vi "FlyWheelSim_Example.vi"() -> ()   [LabVIEW 2019]
uses:
  <vilib>/Rock Robotics/WPI/ThirdParty/JAS_Junk/TrajLib/TypeDef/DCMOTOR.CTL
  <vilib>/Rock Robotics/WPI/ThirdParty/JAS_Junk/TrajLib/TypeDef/LINEAR_SYSTEM.ctl
  <vilib>/Analysis/Matrix/Datatypes/RealMatrix.ctl
  <vilib>/Rock Robotics/WPI/ThirdParty/JAS_Junk/TrajLib/TypeDef/LINEAR_QUADRATIC_REGULATOR.ctl
  <vilib>/Rock Robotics/WPI/ThirdParty/JAS_Junk/TrajLib/TypeDef/KALMAN_FILTER.ctl
  <vilib>/Rock Robotics/WPI/ThirdParty/JAS_Junk/TrajLib/TypeDef/LINEAR_SYSTEM_LOOP.ctl
  <vilib>/Rock Robotics/WPI/ThirdParty/JAS_Junk/TrajLib/TypeDef/LINEAR_PLANT_INV_FF.ctl
  <vilib>/Rock Robotics/WPI/ThirdParty/JAS_Junk/TrajLib/TypeDef/FLYWHEEL_SIM.ctl
  <vilib>/Rock Robotics/WPI/ThirdParty/JAS_Junk/TrajLib/TypeDef/LINEAR_SYSTEM_SIM.ctl
  <vilib>/Rock Robotics/WPI/ThirdParty/JAS_Junk/TrajLib/Enum/DCMOTOR_TYPES_ENUM.ctl
  <vilib>/Rock Robotics/WPI/ThirdParty/JAS_Junk/TrajLib/DCMotor_GetCIM.vi
  <vilib>/Rock Robotics/WPI/ThirdParty/JAS_Junk/TrajLib/DCMotor_GetAndymark9015.vi
  <vilib>/Rock Robotics/WPI/ThirdParty/JAS_Junk/TrajLib/DCMotor_GetAndymarkRs775_125.vi
  <vilib>/Rock Robotics/WPI/ThirdParty/JAS_Junk/TrajLib/DCMotor_GetBag.vi
  <vilib>/Rock Robotics/WPI/ThirdParty/JAS_Junk/TrajLib/DCMotor_GetBanebotsRs550.vi
  <vilib>/Rock Robotics/WPI/ThirdParty/JAS_Junk/TrajLib/DCMotor_GetBanebotsRs775.vi
  <vilib>/Rock Robotics/WPI/ThirdParty/JAS_Junk/TrajLib/DCMotor_GetFalcon500.vi
  <vilib>/Rock Robotics/WPI/ThirdParty/JAS_Junk/TrajLib/DCMotor_GetMiniCIM.vi
  <vilib>/Rock Robotics/WPI/ThirdParty/JAS_Junk/TrajLib/DCMotor_GetNEO.vi
  <vilib>/Rock Robotics/WPI/ThirdParty/JAS_Junk/TrajLib/DCMotor_GetNEO550.vi
  <vilib>/Rock Robotics/WPI/ThirdParty/JAS_Junk/TrajLib/DCMotor_GetRomiBuiltIn.vi
  <vilib>/Rock Robotics/WPI/ThirdParty/JAS_Junk/TrajLib/DCMotor_GetVex775Pro.vi
  <vilib>/Rock Robotics/WPI/ThirdParty/JAS_Junk/TrajLib/MatBuilder_Create.vi
  <vilib>/Rock Robotics/WPI/ThirdParty/JAS_Junk/TrajLib/LinearSystem_New.vi
  <vilib>/Rock Robotics/WPI/ThirdParty/JAS_Junk/TrajLib/MatrixHelper_Zero.vi
  <vilib>/Rock Robotics/WPI/ThirdParty/JAS_Junk/TrajLib/MatBuilder_Fill.vi
  <vilib>/Rock Robotics/WPI/ThirdParty/JAS_Junk/TrajLib/Matrix_Ident.vi
  <vilib>/Rock Robotics/WPI/ThirdParty/JAS_Junk/TrajLib/DCMotor_New.vi
  <vilib>/Rock Robotics/WPI/ThirdParty/JAS_Junk/TrajLib/MatrixHelper_CoerceSize.vi
  <vilib>/Analysis/7linalg.llb/Create Special Matrix.vi
  <vilib>/Analysis/7linalg.llb/Create Special Real Matrix.vi
  <vilib>/Rock Robotics/WPI/ThirdParty/JAS_Junk/TrajLib/Trajectory_Library.lvlib
  <vilib>/Analysis/Matrix/NI_Matrix.lvlib
panel:
  in  "Tab Control":T1(tab)
  out "Motor Current":dbl format="%20.3f"
  out "Battery Voltage":dbl format="%20.3f"
  in  "Shoot ball":bool
  out "CO Chart":cluster{dbl, "Voltage":dbl}(graph)
  in  "Shooter On/Off":bool
  out "Encoer Speed\nRad/Sec":dbl(slide) scale=0.0..300.0
  out "Speed":dbl format="%20.3f"
  out "Cor Err":bool
  out "Kalman Filtered\nSpeed":dbl format="%20.3f"
  out "PV Chart":T2(graph)
  out "Predict Err":bool
  out "Motor Volt Dmd (CO)":dbl format="%20.3f"
  out "shoot Start":bool
  out "Shoot Done":bool
  out "Shooter Motor":T3 {"Jr_KgM2" format="%13.5p"; "L_H" format="%13.5p"; "Kt_NMPerAmp" format="%13.5p"; "KvINV_RadPerSecPerVolt" format="%13.5p"; "R_Ohms" format="%13.5p"; "FreeSpeed_RadPerSec" format="%13.5p"; "FreeCurrent_Amps" format="%13.5p"; "StallCurrent_Amps" format="%13.5p"; "StallTorque_NM" format="%13.5p"; "nominalVoltage_Volts" format="%13.5p"}
  out "m_flywheelPlant_ALT":T4
  out "m_FlyWheelSim":T6 {"GearBox"."Jr_KgM2" format="%13.5p"; "GearBox"."L_H" format="%13.5p"; "GearBox"."Kt_NMPerAmp" format="%13.5p"; "GearBox"."KvINV_RadPerSecPerVolt" format="%13.5p"; "GearBox"."R_Ohms" format="%13.5p"; "GearBox"."FreeSpeed_RadPerSec" format="%13.5p"; "GearBox"."FreeCurrent_Amps" format="%13.5p"; "GearBox"."StallCurrent_Amps" format="%13.5p"; "GearBox"."StallTorque_NM" format="%13.5p"; "GearBox"."nominalVoltage_Volts" format="%13.5p"}
  out "Shooting A":T5
  out "Shooting B":T5
  out "KalmanFilter":T8
  out "Kalman Error":errorcluster
  out "LinearQuadraticRegulator":T9
  out "LQR Error":bool
  out "Linear System Loop":T10
  out "LinSysLoop_Error":bool
  # "<States,States>"
  # "<States,Inputs>"
  # "<Outputs,States>"
  # "<Outputs,Inputs>"
  # "<States, 1>"
  # "<Outputs, 1>"
  # "<Inputs, 1>"
  # "<Outputs, 1>"
  # "<States,States>"
  # "<States,Inputs>"
  # "<Outputs,States>"
  # "<Outputs,Inputs>"
  # "Steady State Gain  \n<States,Outputs>"
  # "State Estimate <Statess,1>"
  # "<States,States>"
  # "<States,Inputs>"
  # "<Outputs,States>"
  # "<Outputs,Inputs>"
  # "Ref State <States,1>"
  # "Comp and capped \noutput <Inputs,1>"
  # "Controller gain\n<Inputs,States>"
  # "<States,1>"
  # "<FUTURE --- CLAMP TYPE -- For now\nuse Normalize>"
  # "Steady State Gain  \n<States,Outputs>"
  # "State Estimate <Statess,1>"
  # "<States,States>"
  # "<States,Inputs>"
  # "<Outputs,States>"
  # "<Outputs,Inputs>"
  # "<States,1>"
  # "<Inputs,1>"
  # "<States,Inputs>"
  # "<States,States>"
  # "Ref State <States,1>"
  # "Comp and capped \noutput <Inputs,1>"
  # "Controller gain\n<Inputs,States>"
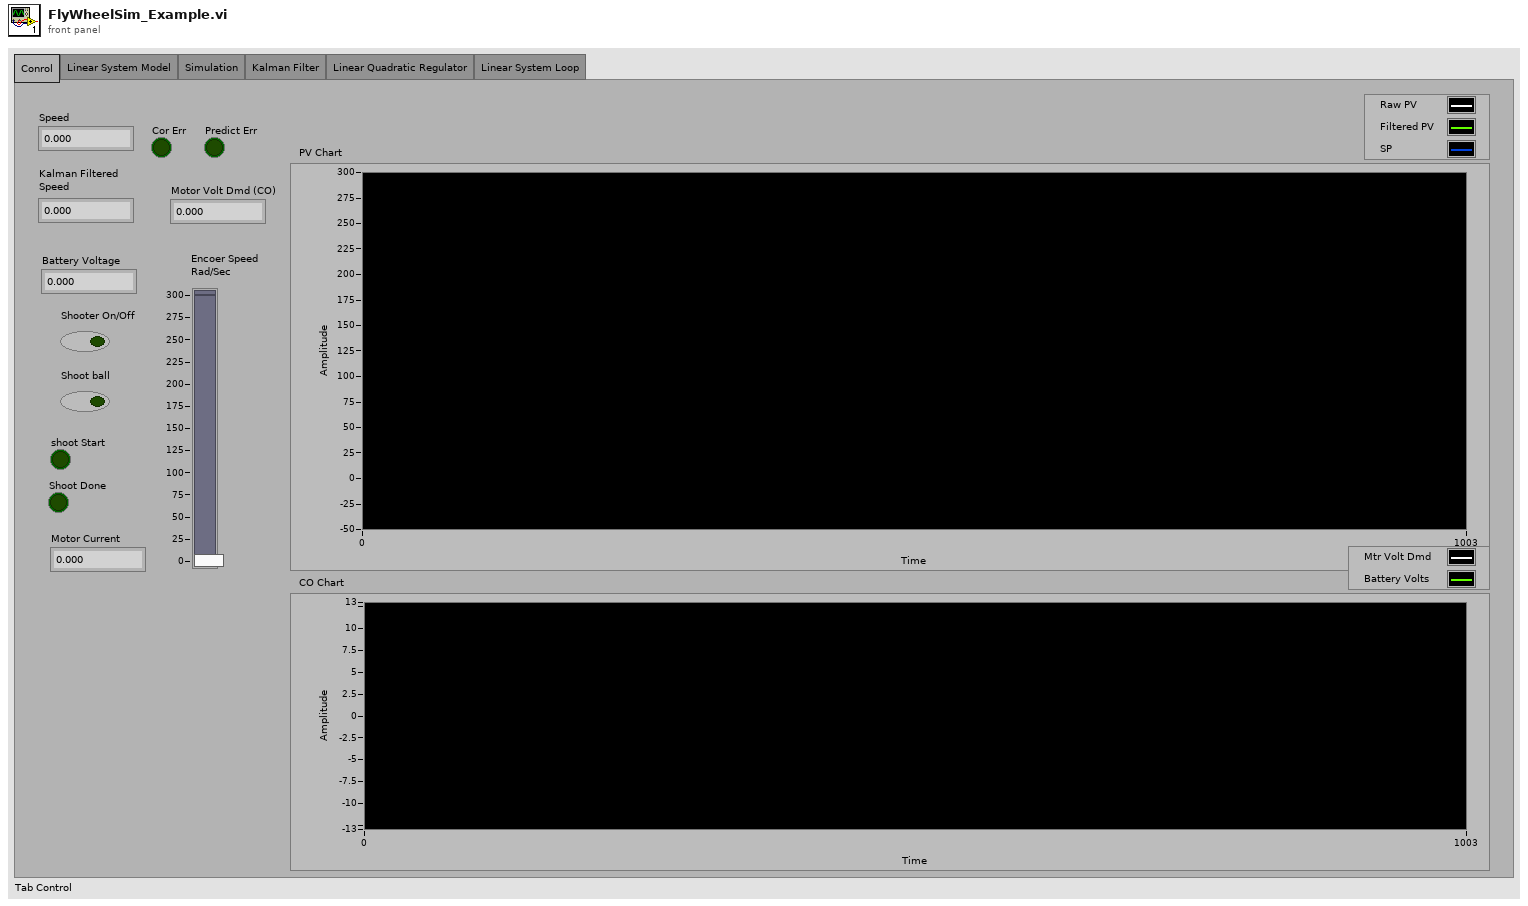
[diagram p1: front panel]
types:
  T1 = enum32{"Conrol", "Linear System Model", "Simulation", "Kalman Filter", "Linear Quadratic Regulator", "Linear System Loop"}
  T2 = cluster{"upper limit":dbl, "Real Matrix Element":dbl, "Real Matrix Element":dbl}
  T3 = typedef "Trajectory_Library.lvlib/DCMOTOR.CTL" = cluster{"nominalVoltage_Volts":dbl, "StallTorque_NM":dbl, "StallCurrent_Amps":dbl, "FreeCurrent_Amps":dbl, "FreeSpeed_RadPerSec":dbl, "R_Ohms":dbl, "KvINV_RadPerSecPerVolt":dbl, "Kt_NMPerAmp":dbl, "L_H":dbl, "Jr_KgM2":dbl}
  T4 = typedef "Trajectory_Library.lvlib/LINEAR_SYSTEM.ctl" = cluster{"m_A":T5, "m_B":T5, "m_C":T5, "m_D":T5, "States":i32, "Inputs":i32, "Outputs":i32}
  T5 = typedef "NI_Matrix.lvlib/RealMatrix.ctl" = dbl[][]
  T6 = typedef "Trajectory_Library.lvlib/FLYWHEEL_SIM.ctl" = cluster{"LinearSystemSim":T7, "GearBox":T3, "Gearing":dbl}
  T7 = typedef "Trajectory_Library.lvlib/LINEAR_SYSTEM_SIM.ctl" = cluster{"m_Plant":T4, "m_X":T5, "m_Y":T5, "m_U":T5, "MeasureStdDev":T5}
  T8 = typedef "Trajectory_Library.lvlib/KALMAN_FILTER.ctl" = cluster{"m_K":T5, "m_xHat":T5, "States":i32, "Outputs":i32, "m_Plant":T4}
  T9 = typedef "Trajectory_Library.lvlib/LINEAR_QUADRATIC_REGULATOR.ctl" = cluster{"m_r":T5, "m_U":T5, "m_K":T5, "States":i32, "Inputs":i32}
  T10 = typedef "Trajectory_Library.lvlib/LINEAR_SYSTEM_LOOP.ctl" = cluster{"Controller":T9, "FeedForward":T11, "Observer":T8, "Next_R":T5, "Clamp Max":T5}
  T11 = typedef "Trajectory_Library.lvlib/LINEAR_PLANT_INV_FF.ctl" = cluster{"m_R":T5, "m_Uff":T5, "m_B":T5, "m_A":T5, "States":i32, "Inputs":i32}
  T12 = typedef "Trajectory_Library.lvlib/DCMOTOR_TYPES_ENUM.ctl" = enum16{"CIM", "AndyMark 9015", "Andy Mark RS 775 125", "Bag", "BaneBots RS 550", "BaneBots RS 775", "Falcon 500", "Mini CIM", "NEO", "NEO 550", "Romi BuiltIn", "Vex 775 Pro"}
  T13 = cluster{"Velocity_RadPerSec":dbl, "Real Matrix Element":dbl, "Real Matrix Element":dbl}
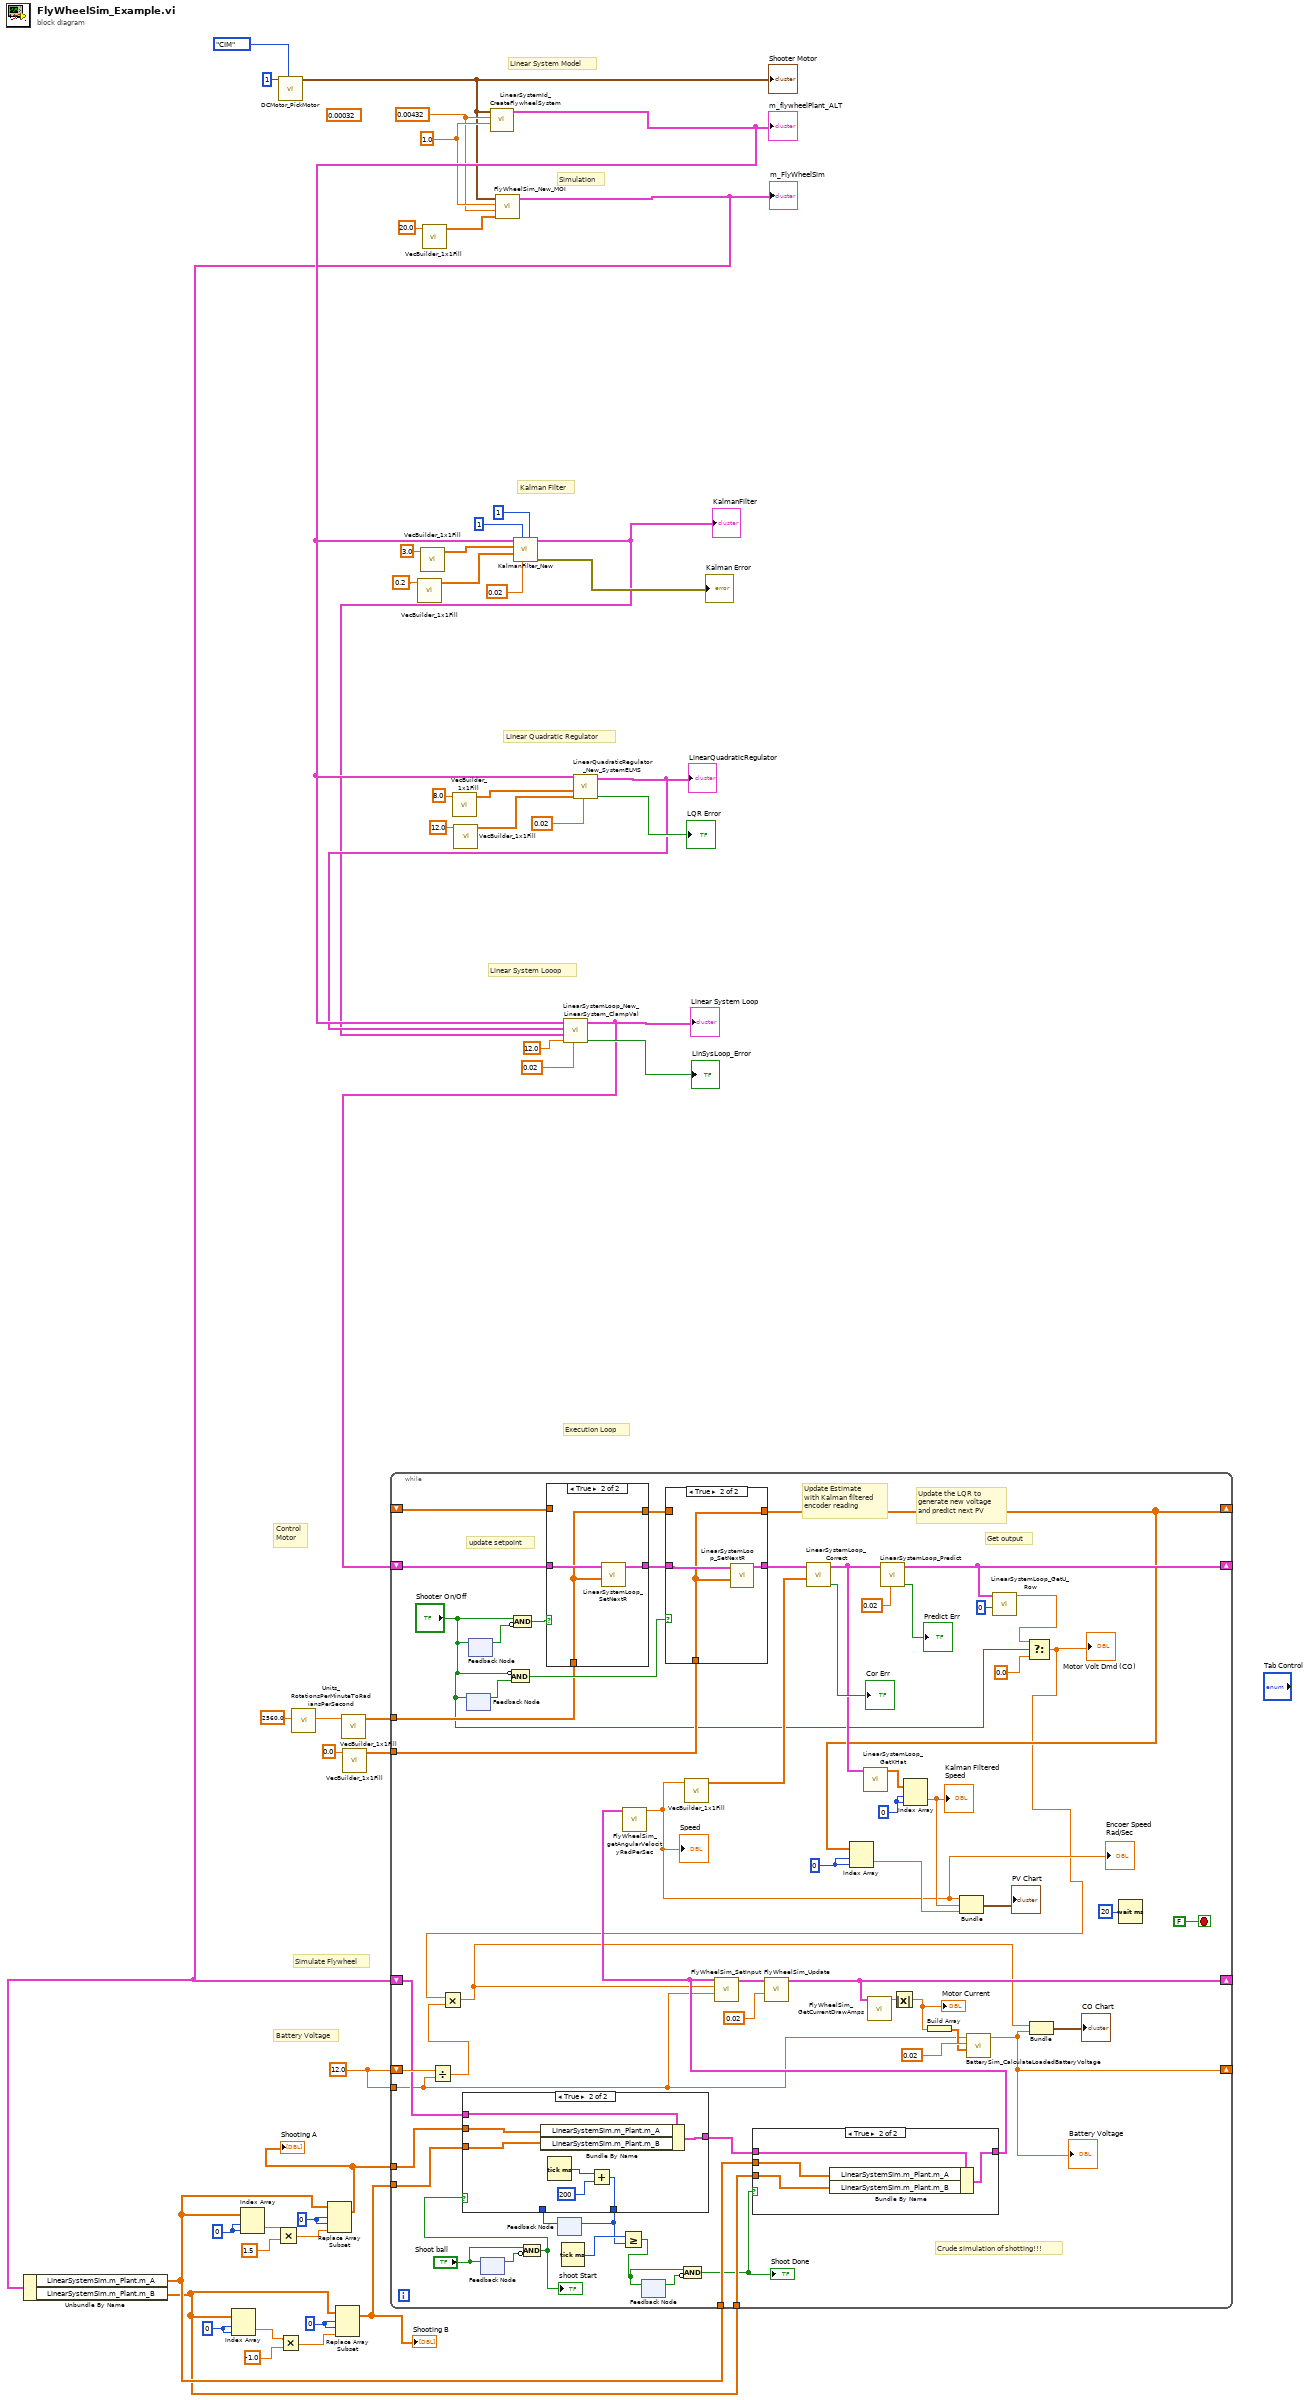
[diagram p0: block diagram]
diagram:
  w14 = 0 ("index (row)")
  w15 = 0 ("index (row)")
  w16 = 0 ("index (row)")
  w17 = 0 ("index (row)")
  w19 = 12.0
  w20 = 0.00432 ("jKgMetersSquared")
  w23 = 1.0 ("G")
  (unwired) 0.00032 ("jKgMetersSquared")
  # "Execution Loop"
  # "Linear System Looop"
  # "Linear Quadratic Regulator"
  # "Kalman Filter"
  # "Simulation"
  # "Linear System Model"
  # "Control\nMotor"
  # "Simulate Flywheel"
  # "Battery Voltage"
  n1 = call <vilib>:"DCMotor_PickMotor.vi"("DCMOTOR_TYPES"=DCMOTOR_TYPES_ENUM."CIM", "Num Motors"=1) -> ("DCMOTOR"=w1:T3)  [unwired: 9 in]
  "Shooter Motor" <- w1
  n2 = call <vilib>:"Units_RotationsPerMinuteToRadiansPerSecond.vi"("RotationsPerMinute"=2560.0) -> ("RadiansPerSecond"=w27:dbl)  [unwired: 10 in]
  n3 = call <vilib>:"VecBuilder_1x1Fill.vi"("R0_C0"=w27) -> ("output matrix"=w25:T5)  [unwired: 10 in]
  n4 = call <vilib>:"VecBuilder_1x1Fill.vi"("R0_C0"=0.0) -> ("output matrix"=w24:T5)  [unwired: 10 in]
  n5 = call <vilib>:"VecBuilder_1x1Fill.vi"("R0_C0"=0.2) -> ("output matrix"=w37:T5)  [unwired: 10 in]
  n6 = call <vilib>:"VecBuilder_1x1Fill.vi"("R0_C0"=3.0) -> ("output matrix"=w38:T5)  [unwired: 10 in]
  n7 = call <vilib>:"VecBuilder_1x1Fill.vi"("R0_C0"=20.0) -> ("output matrix"=w22:T5)  [unwired: 10 in]
  n8 = call <vilib>:"VecBuilder_1x1Fill.vi"("R0_C0"=8.0) -> ("output matrix"=w46:T5)  [unwired: 10 in]
  n9 = call <vilib>:"VecBuilder_1x1Fill.vi"("R0_C0"=12.0) -> ("output matrix"=w44:T5)  [unwired: 10 in]
  n10 = call <vilib>:"LinearSystemId_CreateFlywheelSystem.vi"("G"=w23, "jKgMetersSquared"=w20, "DCMOTOR"=w1) -> ("Linearsystem"=w35:T4)  [unwired: 7 in, 1 out]
  "m_flywheelPlant_ALT" <- w35
  n11 = call <vilib>:"FlyWheelSim_New_MOI.vi"("MeasurementStdDev"=w22, "jKgMetersSquared"=w20, "Gearing"=w23, "GearBox"=w1) -> ("FlyWheelSim"=w18:T6)  [unwired: 6 in, 1 out]
  "m_FlyWheelSim" <- w18
  n12 = Unbundle By Name(w18) -> ("LinearSystemSim.m_Plant.m_A"=w7:T5, "LinearSystemSim.m_Plant.m_B"=w6:T5)
  n13 = Index Array(array=w6, index (row)=w17, index (col)=w17) -> (element=w9:dbl)
  n14 = Index Array(array=w7, index (row)=w16, index (col)=w16) -> (element=w13:dbl)
  n15 = Multiply(x=w13, y=1.5) -> (x*y=w11:dbl)
  n16 = Multiply(x=w9, y=-1.0) -> (x*y=w8:dbl)
  n17 = Replace Array Subset(array=w7, new element=w11, index (row)=w14, index (col)=w14) -> (w5:T5)
  "Shooting A" <- w5
  n18 = Replace Array Subset(array=w6, new element=w8, index (row)=w15, index (col)=w15) -> (w4:T5)
  "Shooting B" <- w4
  n19 = call <vilib>:"KalmanFilter_New.vi"("States"=1, "dt_Seconds"=0.02, "Outputs"=1, "MeasurementStdDevs"=w37, "StateStdDevs"=w38, "Plant"=w35) -> ("Error"=→"Kalman Error":errorcluster, "KalmanFilter"=w33:T8)  [unwired: 4 in]
  "KalmanFilter" <- w33
  n20 = call <vilib>:"LinearQuadraticRegulator_New_SystemELMS.vi"("dt_Seconds"=0.02, "Relms"=w44, "Qelms"=w46, "LINEARSYSTEM"=w35) -> ("Error"=→"LQR Error":bool, "LinearQuadraticRegulator"=w34:T9)  [unwired: 6 in]
  "LinearQuadraticRegulator" <- w34
  n21 = call <vilib>:"LinearSystemLoop_New_LinearSystem_ClampVal.vi"("dT_Seconds"=0.02, "Max_Voltage"=12.0, "Observer"=w33, "Controller"=w34, "Plant"=w35) -> ("Error"=→"LinSysLoop_Error":bool, "Linear System Loop"=w29:T10)  [unwired: 5 in]
  "Linear System Loop" <- w29
  n22 = while {
    shift-right: [w90] -> _
    shift-left: w29 -> [w104]
    tunnel: w25 -> [w102]
    tunnel: w24 -> [w101]
    shift-right: [w79] -> _
    shift-left: w18 -> [w74]
    shift-right: [w84] -> _
    shift-left: _ -> [w85]
    shift-right: [w75] -> _
    shift-left: w19 -> [w81]
    tunnel: w19 -> [w54]
    tunnel: w7 -> [w69]
    tunnel: w6 -> [w68]
    tunnel: w5 -> [w67]
    tunnel: w4 -> [w66]
    stop <- FALSE stop-if-true
    w83 = 0 ("index (row)")
    w97 = 0 ("index (row)")
    # "Crude simulation of shotting!!!"
    # "Get output"
    # "Update the LQR to \ngenerate new voltage\nand predict next PV"
    # "update setpoint"
    # "Update Estimate\nwith Kalman filtered\nencoder reading"
    n23 = Divide(x=w81, y=w54) -> (x/y=w80:dbl)
    n24 = feedback #1() -> (w107:bool)  [unwired: 1 in]
    n25 = feedback-in #1("Shooter On/Off") -> ()
    n26 = feedback-in #2("Shooter On/Off") -> ()
    n27 = feedback #2() -> (w108:bool)  [unwired: 1 in]
    n28 = feedback-in #3("Shoot ball") -> ()
    n29 = feedback #3() -> (w71:bool)  [unwired: 1 in]
    n30 = Compound Arithmetic op=AND(invert "Shooter On/Off", w107) -> (w105:bool)
    n31 = Compound Arithmetic op=AND("Shooter On/Off", invert w108) -> (w106:bool)
    n32 = Compound Arithmetic op=AND("Shoot ball", invert w71) -> (w70:bool)
    "shoot Start" <- w70
    n33 = case shown="True" w106 {
      tunnel: w104 -> [w131 w133]
      tunnel: [w131 w134] -> w103
      tunnel: w102 -> [_ w132]
      tunnel: [w130 w132] -> w86
      tunnel: w85 -> [w130 _]
      frame False {
      }
      frame True {
        n34 = call <vilib>:"LinearSystemLoop_SetNextR.vi"("R"=w132, "input inear System Loop"=w133) -> ("out Linear System Loop"=w134:T10)  [unwired: 8 in, 1 out]
      }
    }
    n35 = feedback #4() -> (w60:u32)  [unwired: 1 in]
    n36 = case shown="True" w70 {
      tunnel: w74 -> [w117 w124]
      tunnel: [w117 w121] -> w73
      tunnel: w67 -> [_ w123]
      tunnel: w66 -> [_ w122]
      tunnel: [w116 w118] -> w61
      tunnel: w60 -> [w116 _]
      frame False {
      }
      frame True {
        n37 = Bundle By Name(cluster=w124, "LinearSystemSim.m_Plant.m_A"=w123, "LinearSystemSim.m_Plant.m_B"=w122) -> (w121:T6)
        n38 = Tick Count (ms)() -> (millisecond timer value=w120:u32)
        n39 = Add(x=w120, y=u32 200) -> (x+y=w118:u32)
      }
    }
    n40 = feedback-in #4(w61) -> ()
    n41 = Tick Count (ms)() -> (millisecond timer value=w65:u32)
    n42 = Greater Or Equal?(x=w65, y=w61) -> (x >= y?=w63:bool)
    n43 = feedback #5() -> (w64:bool)  [unwired: 1 in]
    n44 = feedback-in #5(w63) -> ()
    n45 = case shown="True" w105 {
      tunnel: w103 -> [w126 w128]
      tunnel: [w126 w129] -> w100
      tunnel: w101 -> [_ w127]
      tunnel: w86 -> [w125 _]
      tunnel: [w125 w127] -> w84
      frame False {
      }
      frame True {
        n46 = call <vilib>:"LinearSystemLoop_SetNextR.vi"("R"=w127, "input inear System Loop"=w128) -> ("out Linear System Loop"=w129:T10)  [unwired: 8 in, 1 out]
      }
    }
    n47 = Compound Arithmetic op=AND(w63, invert w64) -> (w62:bool)
    "Shoot Done" <- w62
    n48 = case shown="True" w62 {
      tunnel: w73 -> [w111 w115]
      tunnel: [w111 w114] -> w57
      tunnel: w69 -> [_ w113]
      tunnel: w68 -> [_ w112]
      frame False {
      }
      frame True {
        n49 = Bundle By Name(cluster=w115, "LinearSystemSim.m_Plant.m_A"=w113, "LinearSystemSim.m_Plant.m_B"=w112) -> (w114:T6)
      }
    }
    n50 = call <vilib>:"FlyWheelSim_getAngularVelocityRadPerSec.vi"("FlyWheelSim"=w57) -> ("Velocity_RadPerSec"=w56:dbl)  [unwired: 10 in]
    "Encoer Speed\nRad/Sec" <- w56
    "Speed" <- w56
    n51 = call <vilib>:"VecBuilder_1x1Fill.vi"("R0_C0"=w56) -> ("output matrix"=w99:T5)  [unwired: 10 in]
    n52 = call <vilib>:"LinearSystemLoop_Correct.vi"("Y"=w99, "input inear System Loop"=w100) -> ("Error"=→"Cor Err":bool, "out Linear System Loop"=w93:T10)  [unwired: 8 in]
    n53 = Index Array(array=w84, index (row)=w83, index (col)=w83) -> (element=w82:dbl)
    n54 = call <vilib>:"LinearSystemLoop_GetXHat.vi"("input inear System Loop"=w93) -> ("XHat"=w96:T5)  [unwired: 10 in]
    n55 = call <vilib>:"LinearSystemLoop_Predict.vi"("dT_Seconds"=0.02, "input inear System Loop"=w93) -> ("Error"=→"Predict Err":bool, "out Linear System Loop"=w90:T10)  [unwired: 8 in]
    n56 = Index Array(array=w96, index (row)=w97, index (col)=w97) -> (element=w95:dbl)
    "Kalman Filtered\nSpeed" <- w95
    n57 = Bundle("Velocity_RadPerSec"=w56, "Real Matrix Element"=w95, "Real Matrix Element"=w82) -> (→"PV Chart":T13)  [unwired: 1 in]
    n58 = call <vilib>:"LinearSystemLoop_GetU_Row.vi"("Row"=0, "input inear System Loop"=w90) -> ("U"=w53:dbl)  [unwired: 9 in]
    n59 = Select(t=w53, s="Shooter On/Off", f=0.0) -> (s? t:f=w52:dbl)
    "Motor Volt Dmd (CO)" <- w52
    n60 = Multiply(x=w52, y=w80) -> (x*y=w55:dbl)
    n61 = call <vilib>:"FlyWheelSim_SetInput.vi"("Battery_Volts"=w54, "Volts"=w55, "FlyWheelSim"=w57) -> ("out FlyWheelSim"=w88:T6)  [unwired: 8 in]
    n62 = call <vilib>:"FlyWheelSim_Update.vi"("dT_Seconds"=0.02, "FlyWheelSim"=w88) -> ("out FlyWheelSim"=w79:T6)  [unwired: 8 in, 1 out]
    n63 = call <vilib>:"FlyWheelSim_GetCurrentDrawAmps.vi"("FlyWheelSim"=w79) -> ("Current_Amps"=w59:dbl)  [unwired: 10 in]
    n64 = Absolute Value(x=w59) -> (abs(x)=w58:dbl)
    "Motor Current" <- w58
    n65 = Build Array(w58) -> (w77:dbl[])
    n66 = call <vilib>:"BatterySim_CalculateLoadedBatteryVoltage.vi"("Currents"=w77, "Resistance_Ohms"=0.02, "NominalVoltage"=w54) -> ("Voltage"=w75:dbl)  [unwired: 8 in]
    "Battery Voltage" <- w75
    n67 = Bundle(w55, "Voltage"=w75) -> (→"CO Chart":cluster{dbl, "Voltage":dbl})  [unwired: 1 in]
    n68 = Wait (ms)(milliseconds to wait=u32 20) -> ()  [unwired: 1 out]
  }
